vi "Run RegExp.vi"(6 "submatches? (T)":bool=TRUE, 7 "flags":T1, 8 "error in (no error)":errorcluster, 9 "offset (0)":i32, 10 "regular expression":string, 11 "string":string) -> (0 "error out":errorcluster, 1 "offset past match":i32, 2 "after match":string, 3 "before match":string, 4 "matches":string[](array[string]))   [LabVIEW 2020, in "Stream.lvlib" / "URLPattern.lvclass"]
uses:
  URLPattern.lvclass
  RegExp Flags.ctl
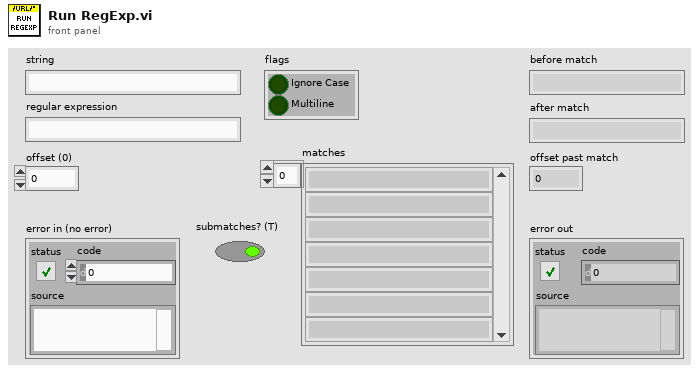
[diagram p1: front panel]
types:
  T1 = typedef "Stream.lvlib/URLPattern.lvclass/RegExp Flags.ctl" = cluster{"Ignore Case":bool, "Multiline":bool}
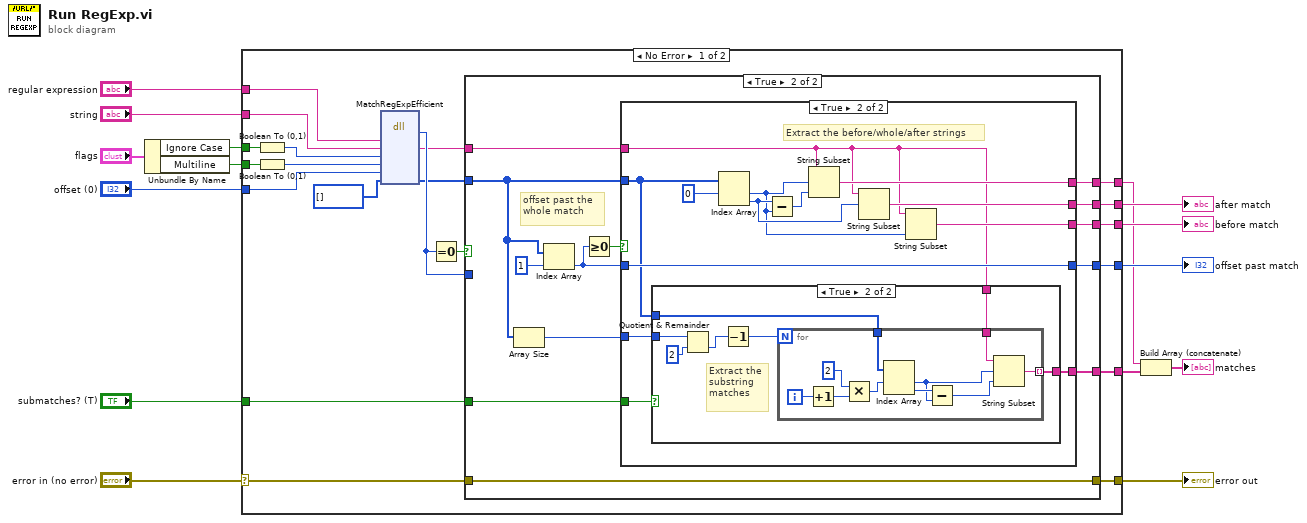
[diagram p0: block diagram]
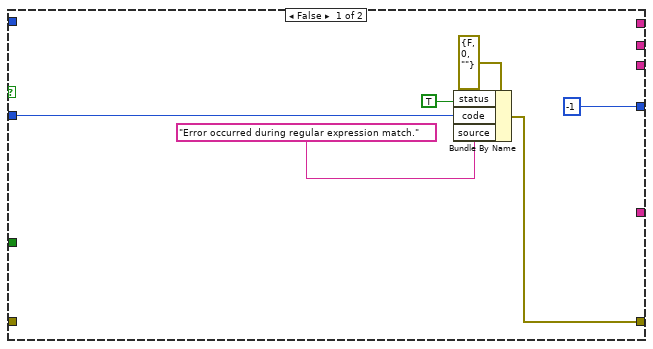
[diagram p2: hidden frame]
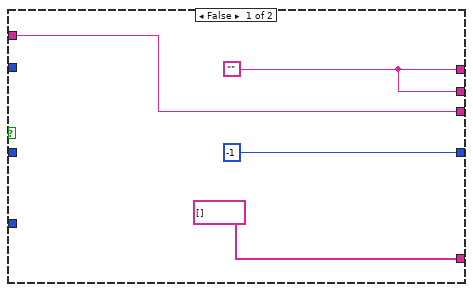
[diagram p3: hidden frame]
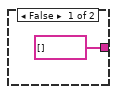
[diagram p4: hidden frame]
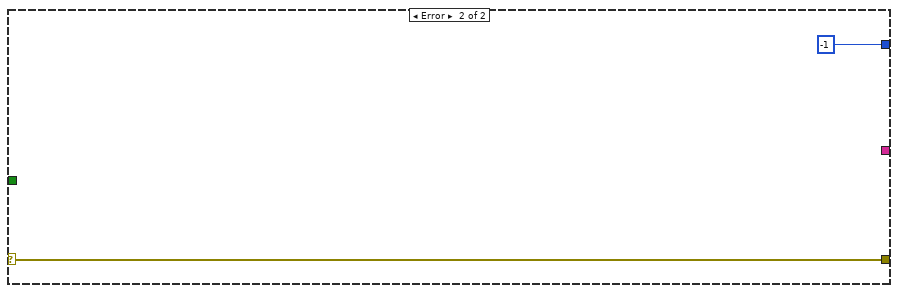
[diagram p5: hidden frame]
diagram:
  n1 = Unbundle By Name("flags") -> ("Ignore Case"=w2:bool, "Multiline"=w1:bool)
  n2 = case shown="No Error" "error in (no error)" {
    selector: "error in (no error)" -> [w26 w91]
    tunnel: "regular expression" -> [w28 _]
    tunnel: "string" -> [w29 _]
    tunnel: w2 -> [w35 _]
    tunnel: w1 -> [w34 _]
    tunnel: "offset (0)" -> [w32 _]
    tunnel: [w25 w91] -> w11
    tunnel: [w21 _] -> w5
    tunnel: [w20 _] -> w10
    tunnel: [w19 _] -> w9
    tunnel: [w18 -1] -> w8
    tunnel: [w17 _] -> w7
    tunnel: "submatches? (T)" -> [w16 _]
    frame No Error {
      n3 = Boolean To (0,1)(Boolean=w35) -> (0, 1=w30:i16)
      n4 = Boolean To (0,1)(Boolean=w34) -> (0, 1=w31:i16)
      n5 = dll-call lib="LabVIEW" fn="MatchRegExpEfficient"("regexp"=w28, "subject"=w29, "noCase"=w30, "multiline"=w31, "offsetIn"=w32, "offsetsOut"=i32[] []) -> ("return type"=w24:i32, "subject"=w22:string, "offsetsOut"=w23:i32[])  [unwired: 7 in, 2 out]
      n6 = Equal To 0?(x=w24) -> (x = 0?=w27:bool)
      n7 = case shown="True" w27 {
        tunnel: w24 -> [w37 _]
        tunnel: w26 -> [_ w54]
        tunnel: [w38 w54] -> w25
        tunnel: w23 -> [_ w50]
        tunnel: w22 -> [_ w48]
        tunnel: [_ w47] -> w21
        tunnel: [_ w46] -> w20
        tunnel: [_ w45] -> w19
        tunnel: [-1 w44] -> w18
        tunnel: [_ w43] -> w17
        tunnel: w16 -> [_ w42]
        frame False {
          n8 = Bundle By Name(cluster=errorcluster {"status"=FALSE, "code"=0, "source"=""} ("error in (no error)"), "status"=TRUE, "code"=w37, "source"="Error occurred during regular expression match.") -> (w38:errorcluster)
        }
        frame True {
          # "offset past the whole match"
          n9 = Array Size(array=w50) -> (size(s)=w52:i32)
          n10 = Index Array(array=w50, index=1) -> (element=w51:i32)
          n11 = Greater Or Equal To 0?(x=w51) -> (x >= 0?=w49:bool)
          n12 = case shown="True" w49 {
            tunnel: [string[] [] w71] -> w43
            tunnel: w48 -> [w55 w61]
            tunnel: [w56 w68] -> w47
            tunnel: w50 -> [_ w66]
            tunnel: w52 -> [_ w60]
            tunnel: [-1 w67] -> w44
            tunnel: w51 -> [_ w67]
            tunnel: [w56 w63] -> w46
            tunnel: [w55 w62] -> w45
            tunnel: w42 -> [_ w59]
            frame False {
              w56 = ""
            }
            frame True {
              # "Extract the before/whole/after strings"
              n13 = case shown="True" w59 {
                tunnel: [string[] [] w79] -> w71
                tunnel: w66 -> [_ w78]
                tunnel: w61 -> [_ w77]
                tunnel: w60 -> [_ w76]
                frame False {
                }
                frame True {
                  # "Extract the substring matches"
                  n14 = Quotient & Remainder(x=w76, y=2) -> (floor(x/y)=w74:i32)  [unwired: 1 out]
                  n15 = Decrement(x=w74) -> (x-1=w73:i32)
                  n16 = for {
                    N: w73 -> [_]
                    tunnel: w78 -> [w83]
                    tunnel: w77 -> [w84]
                    tunnel: [w80] -> w79 mode=indexing
                    i -> [w81]
                    n17 = Increment(x=w81) -> (x+1=w89:i32)
                    n18 = Multiply(x=2, y=w89) -> (x*y=w82:i32)
                    n19 = Index Array(array=w83, index #1=w82) -> (element #1=w85:i32, element #2=w86:i32)  [unwired: 1 in]
                    n20 = Subtract(x=w86, y=w85) -> (x-y=w87:i32)
                    n21 = String Subset(string=w84, offset (0)=w85, length (rest)=w87) -> (substring=w80:string)
                  }
                }
              }
              n22 = Index Array(array=w66, index #1=0 ("index")) -> (element #1=w64:i32, element #2=w65:i32)  [unwired: 1 in]
              n23 = Subtract(x=w65, y=w64) -> (x-y=w69:i32)
              n24 = String Subset(string=w61, offset (0)=w64, length (rest)=w69) -> (substring=w68:string)
              n25 = String Subset(string=w61, offset (0)=w65) -> (substring=w63:string)  [unwired: 1 in]
              n26 = String Subset(string=w61, length (rest)=w64) -> (substring=w62:string)  [unwired: 1 in]
            }
          }
        }
      }
    }
    frame Error {
    }
  }
  "before match" <- w9
  "after match" <- w10
  "error out" <- w11
  "offset past match" <- w8
  n27 = Build Array (concatenate)(w5, w7) -> (→"matches":string[])
